vi "Equal.vi"   [LabVIEW 2020, in "NI_Matrix.lvlib"]
doc: "Returns TRUE if <B>x</B> is equal to <B>y</B>. Otherwise, this function returns FALSE."
uses:
  NI_Matrix.lvlib
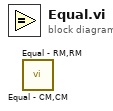
[diagram p0: block diagram]
diagram:
  n1 = call "Equal - CM,CM.vi"() -> ()  [unwired: 2 in, 1 out]
  n2 = call "Equal - RM,RM.vi"() -> ()  [unwired: 2 in, 1 out]
